vi "Main.vi"(11 "Module Admin":refnum<class "Delacor_lib_QMH_Cloneable Module Admin.lvclass">) -> ()   [LabVIEW 2025, in "Data Log.lvlib"]
doc: "This template is based off of the Queued Message Handler design pattern and the Queued Message Handler project template that ships with LabVIEW.\n\nThe main difference is that the queue is private to this module and communication between modules is performed via Broadcast and Request events.\n\nRequest events are wrapped in public API methods and are handled in the Event Handling Loop (EHL) of this VI. Any module can register for Broadcast events sent by this module. The EHL generates messages based on user interface actions.\n\nThe Message Handling Loop (MHL) processes messages generated by the EHL, or by other messages. The messages are string values, so new messages can be added easily to the Message Cases case structure in the MHL. Each message cluster can also provide an optional value for Message Data, which is a variant that can be converted to whatever message-specific data is required.\n_____\nBased on DQMH Dev Tools: Project Template 7.1.2.1547."
uses:
  Data Log.lvlib
  <vilib>/Delacor/Delacor QMH/Libraries/Message Queue_class/Delacor_lib_QMH_Message Queue.lvclass
  Module Data--cluster.ctl
  <vilib>/Utility/miscctls.llb/LVPointTypeDef.ctl
  <vilib>/Delacor/Delacor QMH/Libraries/Message Queue_class/Delacor_lib_QMH_Enqueue Message (Single).vi
  Stop Argument--cluster.ctl
  <vilib>/Delacor/Delacor QMH/Libraries/Cloneable Module Admin_class/Delacor_lib_QMH_Cloneable Module Admin.lvclass
  Write to .csv (Reply Payload)--cluster.ctl
  Write to .csv Argument--cluster.ctl
  Classes/Data Log/Data Log.lvclass
  Append data (Reply Payload)--cluster.ctl
  Append data Argument--cluster.ctl
panel:
  out "error out":errorcluster
  out "Status":string
  in  "Simulate EHL Error":bool
  in  "Simulate MHL Error":bool
  # "Other processes communicate with this Module via its Public API (wrappers for its Request Events).\n\nThis Module communicates with other processes via its Broadcast Events.\nAny process that wants to receive these messages can register for this module's Broadcast events."
  # "This template is for the DQMH framework. See the block diagram for more information on how to use this template."
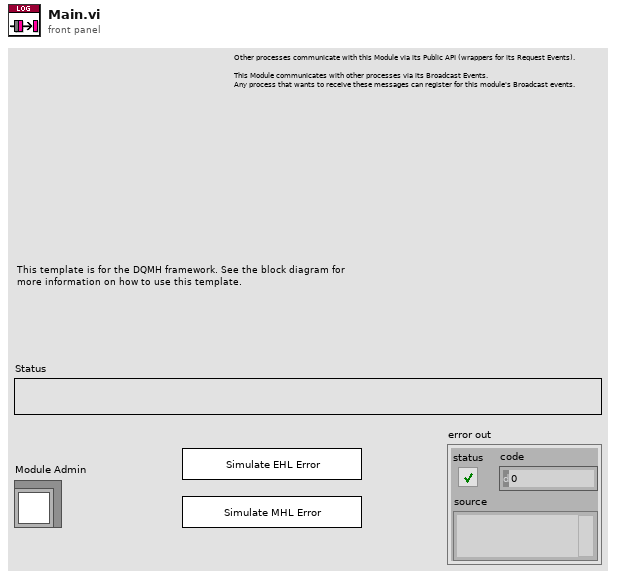
[diagram p1: front panel]
types:
  T1 = typedef "Data Log.lvlib/Request Events--cluster.ctl" = cluster{"Stop Module":refnum<user-event>, "Show Panel":refnum<user-event>, "Hide Panel":refnum<user-event>, "Show Diagram":refnum<user-event>, "Get Module Execution Status":refnum<user-event>, "Write to .csv":refnum<user-event>, "Append data":refnum<user-event>}
  T2 = typedef "Data Log.lvlib/Module Data--cluster.ctl" = cluster{"Status":string, "Data Log Object":refnum<class "Data Log.lvclass">}
  T3 = enum32{"invalid lock state", "Not Locked", "Locked (No Password)", "Password-protected"}
  T4 = typedef "Data Log.lvlib/Stop Argument--cluster.ctl" = cluster{"Module ID":i32, "Origin":string, "Exit via Stop Module Req?":bool, "Wait for Module to stop?":bool}
  T5 = typedef "Data Log.lvlib/Write to .csv Argument--cluster.ctl" = cluster{"Module ID":i32, "csv path":path, "Wait Notifier":refnum<notifier>, "wait for reply":bool}
  T6 = typedef "Data Log.lvlib/Append data Argument--cluster.ctl" = cluster{"Module ID":i32, "Time Stamp":timestamp, "Array":dbl[], "Wait Notifier":refnum<notifier>, "wait for reply":bool}
  T7 = typedef "LVPointTypeDef.ctl" = cluster{"Horizontal":i16, "Vertical":i16}
  T8 = enum32{"Invalid", "Standard", "Closed", "Hidden", "Minimized", "Maximized"}
  T9 = typedef "Data Log.lvlib/Write to .csv (Reply Payload)--cluster.ctl" = cluster{"Module ID":i32, "error":errorcluster}
  T10 = typedef "Data Log.lvlib/Append data (Reply Payload)--cluster.ctl" = cluster{"Module ID":i32, "error":errorcluster}
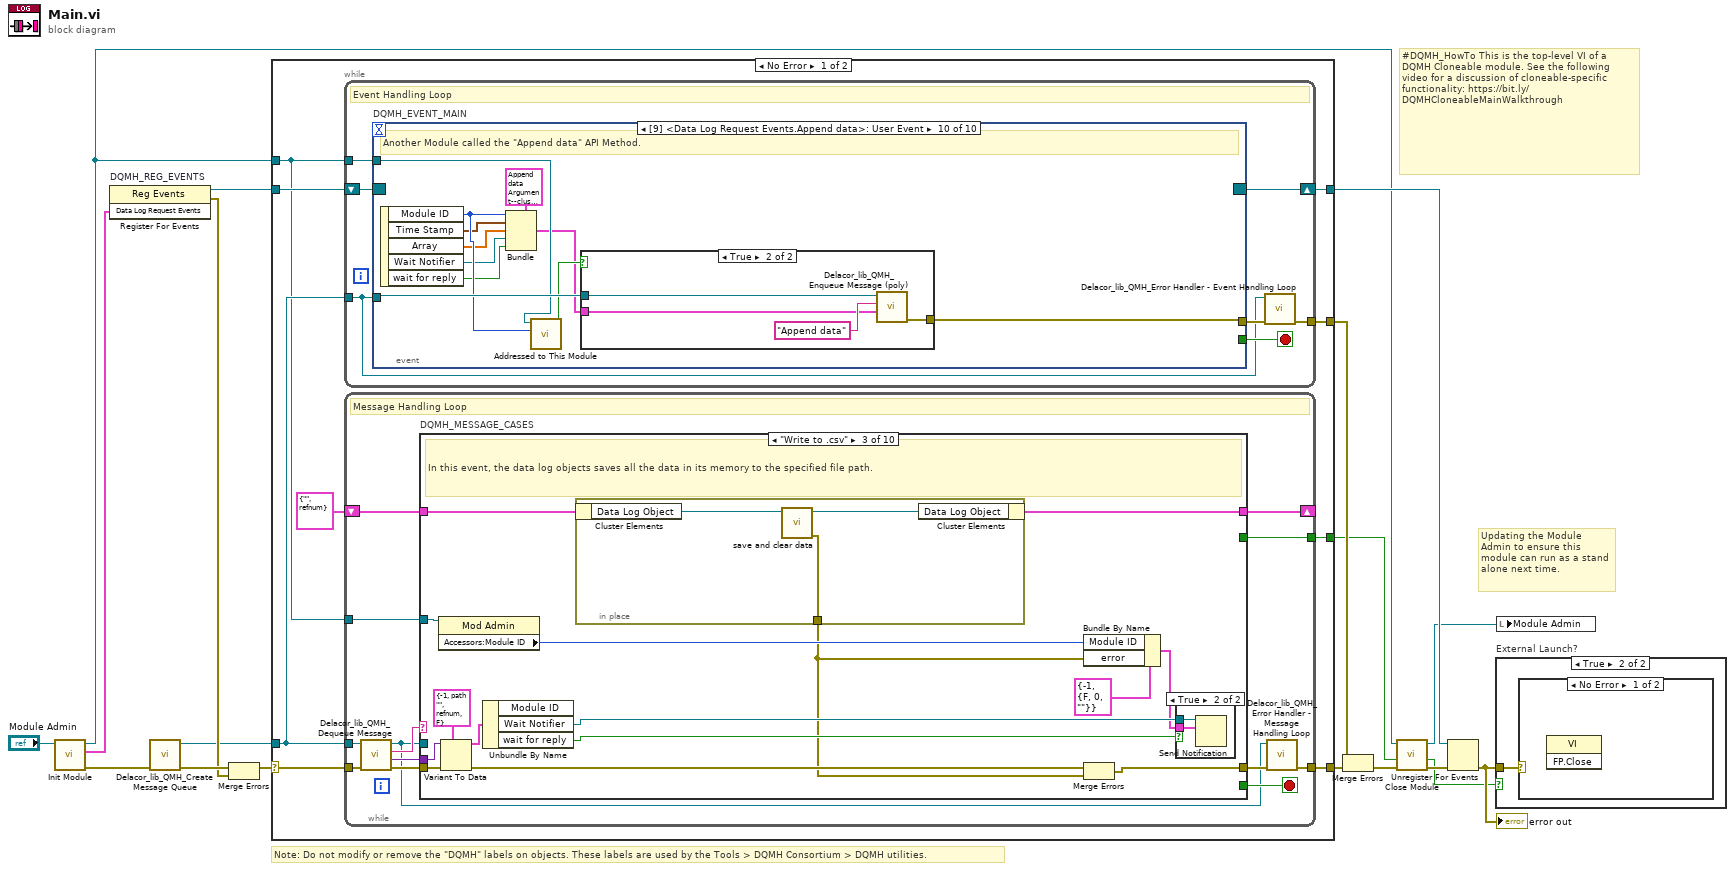
[diagram p0: block diagram]
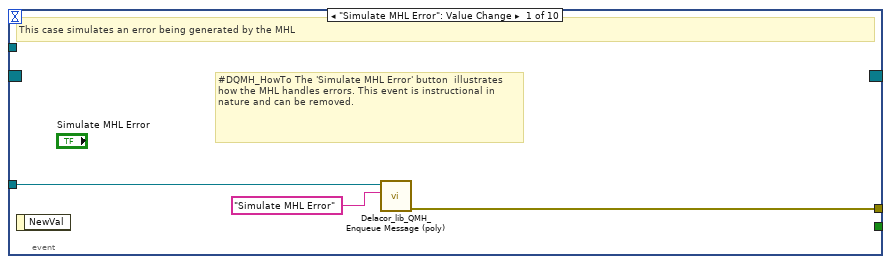
[diagram p2: hidden frame]
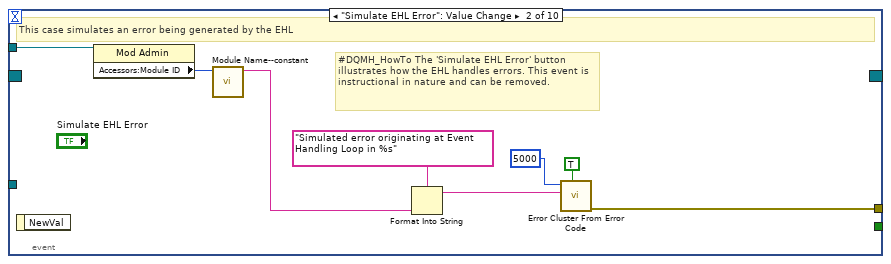
[diagram p3: hidden frame]
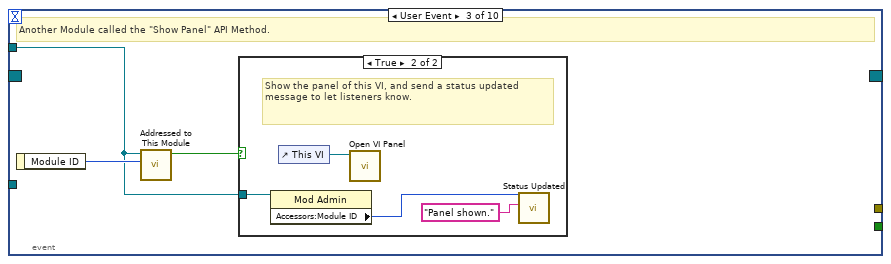
[diagram p4: hidden frame]
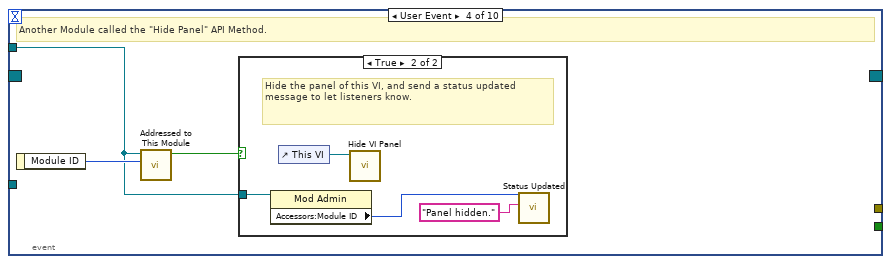
[diagram p6: hidden frame]
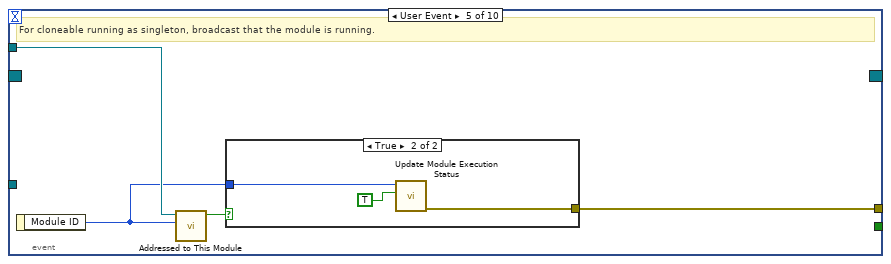
[diagram p8: hidden frame]
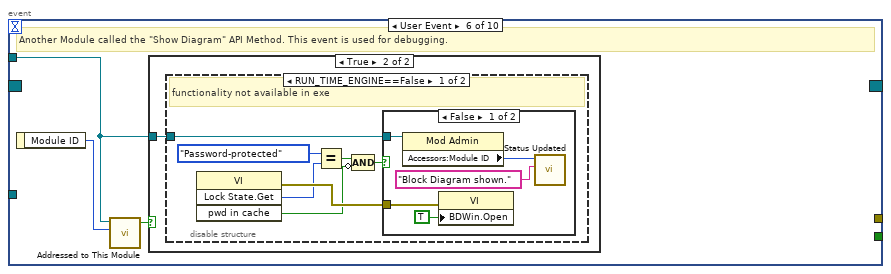
[diagram p10: hidden frame]
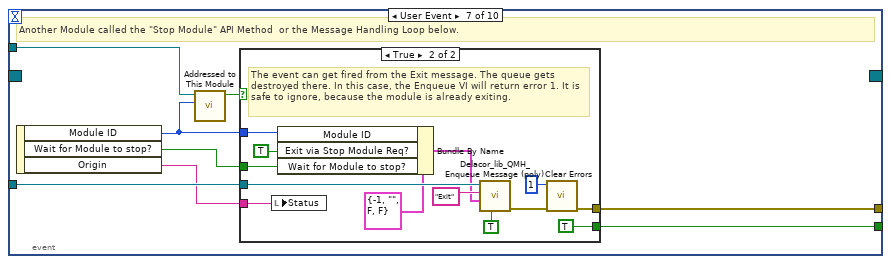
[diagram p14: hidden frame]
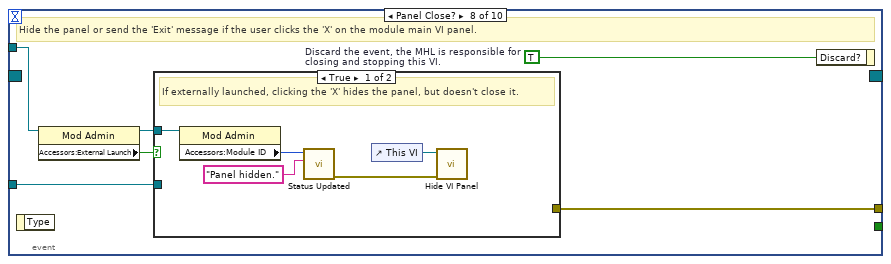
[diagram p16: hidden frame]
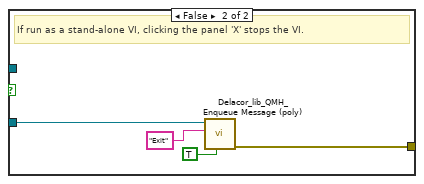
[diagram p17: hidden frame]
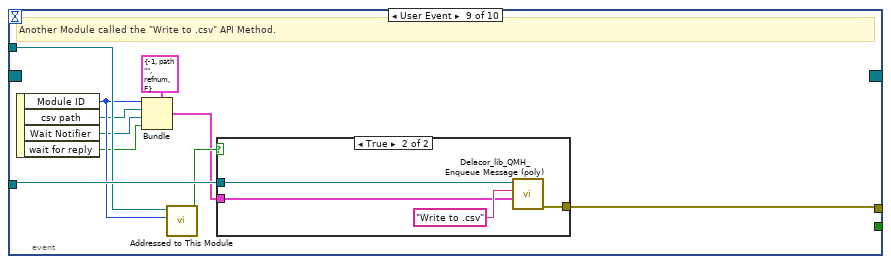
[diagram p18: hidden frame]
diagram:
  # "#DQMH_HowTo This is the top-level VI of a DQMH Cloneable module. See the following video for a discussion of cloneable-specific functionality: https://bit.ly/DQMHCloneableMainWalkthrough"
  # "Note: Do not modify or remove the \"DQMH\" labels on objects. These labels are used by the Tools > DQMH Consortium > DQMH utilities."
  # "Updating the Module Admin to ensure this module can run as a stand alone next time."
  n1 = call "Init Module.vi"("Cloneable Module Admin in"="Module Admin") -> ("error out"=w15:errorcluster, "Data Log Request Events"=w7:T1, "Cloneable Module Admin out"=w4:refnum<class "Delacor_lib_QMH_Cloneable Module Admin.lvclass">)  [unwired: 8 in]
  n2 = register-events "DQMH_REG_EVENTS"(w7) -> (reference out=w8:refnum<event-registration>, error out=w10:errorcluster)  [unwired: 2 in]
  n3 = call <vilib>:"Delacor_lib_QMH_Create Message Queue.vi"("error in"=w15) -> ("error out"=w12:errorcluster, "Message Queue"=w6:refnum<class "Delacor_lib_QMH_Message Queue.lvclass">)  [unwired: 9 in]
  n4 = Merge Errors(w12, w10) -> (w11:errorcluster)
  n5 = case shown="No Error" w11 {
    selector: w11 -> [w25 w300]
    tunnel: [w27 w299] -> w16
    tunnel: [w24 w298] -> w9
    tunnel: w8 -> [w22 w298]
    tunnel: w6 -> [w21 w291]
    tunnel: [w26 _] -> w17
    tunnel: w4 -> [w20 w294]
    tunnel: [w19 _] -> w2
    frame No Error {
      n6 = while {
        tunnel: w21 -> [w28]
        shift-right: [w31] -> w24
        shift-left: w22 -> [w32]
        tunnel: [w33] -> w26
        tunnel: w20 -> [w29]
        stop <- w30 stop-if-true
        # "Event Handling Loop"
        n7 = event "DQMH_EVENT_MAIN" shown="[9] <Data Log Request Events.Append data>: User Event" {
          selector: w32 -> [_ _ _ _ _ _ _ _ _ _]
          dyn-events: [_ _ _ _ _ _ _ _ _ _] -> w31
          timeout: _ -> [_ _ _ _ _ _ _ _ _ _]
          tunnel: [_ _ _ _ _ _ w86 _ _ _] -> w30
          tunnel: w28 -> [w36 _ _ _ _ _ w89 w106 w128 w143]
          tunnel: [w37 w45 _ _ w63 _ w90 w109 w119 w133] -> w34
          tunnel: w29 -> [_ w44 w46 w53 w61 w67 w88 w107 w126 w141]
          event "Simulate MHL Error": Value Change {
            # "#DQMH_HowTo The 'Simulate MHL Error' button  illustrates how the MHL handles errors. This event is instructional in nature and can be removed."
            # "This case simulates an error being generated by the MHL"
            n8 = event-data() -> ()  [unwired: 1 in, 1 out]
            n9 = call-poly <vilib>:"Delacor_lib_QMH_Enqueue Message (poly).vi"("Message"="Simulate MHL Error", "Message Queue in"=w36) -> ("error out"=w37:errorcluster)  [unwired: 8 in, 1 out]
          }
          event "Simulate EHL Error": Value Change {
            # "#DQMH_HowTo The 'Simulate EHL Error' button  illustrates how the EHL handles errors. This event is instructional in nature and can be removed."
            # "This case simulates an error being generated by the EHL"
            n10 = event-data() -> ()  [unwired: 1 in, 1 out]
            n11 = property on="Property Node" class="Mod Admin"(reference=w44) -> ("Accessors:Module ID"=w43:i32)  [unwired: 1 in, 2 out]
            n12 = call "Module Name--constant.vi"("Module ID"=w43) -> ("Module Name"=w38:string)  [unwired: 10 in]
            n13 = Format Into String(format string="Simulated error originating at Event Handling Loop in %s", w38) -> (resulting string=w41:string)  [unwired: 2 in, 1 out]
            n14 = call <vilib>:"Error Cluster From Error Code.vi"("show call chain? (False)"=TRUE, "error message (\"\")"=w41, "error code (0)"=5000) -> ("error out"=w45:errorcluster)  [unwired: 6 in]
          }
          event User Event {
            # "Another Module called the \"Show Panel\" API Method."
            n15 = event-data() -> ("Module ID"=w47:i32)  [unwired: 1 in]
            n16 = call "Addressed to This Module.vi"("Module ID from Argument"=w47, "Module Admin"=w46) -> ("Addressed to this instance?"=w48:bool)  [unwired: 8 in, 1 out]
            n17 = case shown="True" w48 {
              tunnel: w46 -> [_ w50]
              frame False {
              }
              frame True {
                # "Show the panel of this VI, and send a status updated message to let listeners know."
                n18 = property on="Property Node" class="Mod Admin"(reference=w50) -> ("Accessors:Module ID"=w49:i32)  [unwired: 1 in, 2 out]
                n19 = control-ref of="This VI"() -> (w52:refnum<vi>)
                n20 = call "Open VI Panel.vi"("VI"=w52) -> ()  [unwired: 10 in, 1 out]
                n21 = call "Status Updated.vi"("Status"="Panel shown." ("format string"), "Module ID"=w49) -> ()  [unwired: 9 in, 1 out]
              }
            }
          }
          event User Event {
            # "Another Module called the \"Hide Panel\" API Method."
            n22 = event-data() -> ("Module ID"=w54:i32)  [unwired: 1 in]
            n23 = call "Addressed to This Module.vi"("Module ID from Argument"=w54, "Module Admin"=w53) -> ("Addressed to this instance?"=w55:bool)  [unwired: 8 in, 1 out]
            n24 = case shown="True" w55 {
              tunnel: w53 -> [_ w57]
              frame False {
              }
              frame True {
                # "Hide the panel of this VI, and send a status updated message to let listeners know."
                n25 = property on="Property Node" class="Mod Admin"(reference=w57) -> ("Accessors:Module ID"=w56:i32)  [unwired: 1 in, 2 out]
                n26 = control-ref of="This VI"() -> (w59:refnum<vi>)
                n27 = call "Hide VI Panel.vi"("VI"=w59) -> ()  [unwired: 10 in, 1 out]
                n28 = call "Status Updated.vi"("Status"="Panel hidden." ("format string"), "Module ID"=w56) -> ()  [unwired: 9 in, 1 out]
              }
            }
          }
          event User Event {
            # "For cloneable running as singleton, broadcast that the module is running."
            n29 = event-data() -> ("Module ID"=w60:i32)  [unwired: 1 in]
            n30 = call "Addressed to This Module.vi"("Module ID from Argument"=w60, "Module Admin"=w61) -> ("Addressed to this instance?"=w62:bool)  [unwired: 8 in, 1 out]
            n31 = case shown="True" w62 {
              tunnel: [_ w66] -> w63
              tunnel: w60 -> [_ w65]
              frame False {
              }
              frame True {
                n32 = call "Update Module Execution Status.vi"("Running?"=TRUE, "Module ID"=w65) -> ("error out"=w66:errorcluster)  [unwired: 9 in]
              }
            }
          }
          event User Event {
            # "Another Module called the \"Show Diagram\" API Method. This event is used for debugging."
            n33 = event-data() -> ("Module ID"=w68:i32)  [unwired: 1 in]
            n34 = call "Addressed to This Module.vi"("Module ID from Argument"=w68, "Module Admin"=w67) -> ("Addressed to this instance?"=w69:bool)  [unwired: 8 in, 1 out]
            n35 = case shown="True" w69 {
              tunnel: w67 -> [_ w70]
              frame False {
              }
              frame True {
                n36 = disable-structure shown="RUN_TIME_ENGINE==False" {
                  disable-tunnel: w70 -> [w71 _]
                  frame condition #0 (active) {
                    # "functionality not available in exe"
                    n37 = invoke on="Invoke Node" class="VI" method="Lock State.Get"() -> (error out=w77:errorcluster, "Get Lock State"=w76:T3, "pwd in cache"=w73:bool)  [unwired: 4 in, 1 out]
                    n38 = Equal?(x=T3."Password-protected", y=w76) -> (x = y?=w74:bool)
                    n39 = Compound Arithmetic op=AND(w74, invert w73) -> (w72:bool)
                    n40 = case shown="False" w72 {
                      tunnel: w77 -> [w82 _]
                      tunnel: w71 -> [w79 _]
                      frame False {
                        n41 = property on="Property Node" class="Mod Admin"(reference=w79) -> ("Accessors:Module ID"=w78:i32)  [unwired: 1 in, 2 out]
                        n42 = property on="Property Node" class="VI"(error in=w82, "BDWin.Open"=TRUE ("Block Diagram Window:Open")) -> ()  [unwired: 1 in, 2 out]
                        n43 = call "Status Updated.vi"("Status"="Block Diagram shown." ("format string"), "Module ID"=w78) -> ()  [unwired: 9 in, 1 out]
                      }
                      frame True {
                        # "Password-protected VI, and the password is not in the cache. Do not show the diagram."
                      }
                    }
                  }
                  frame condition #1 {
                  }
                }
              }
            }
          }
          event User Event {
            # "Another Module called the \"Stop Module\" API Method  or the Message Handling Loop below."
            n44 = event-data() -> ("Module ID"=w84:i32, "Wait for Module to stop?"=w85:bool, "Origin"=w83:string)  [unwired: 1 in]
            n45 = call "Addressed to This Module.vi"("Module ID from Argument"=w84, "Module Admin"=w88) -> ("Addressed to this instance?"=w87:bool)  [unwired: 8 in, 1 out]
            n46 = case shown="True" w87 {
              tunnel: [_ w102] -> w90
              tunnel: w89 -> [_ w98]
              tunnel: [_ TRUE] -> w86
              tunnel: w85 -> [_ w93]
              tunnel: w84 -> [_ w95]
              tunnel: w83 -> [_ w91]
              frame False {
              }
              frame True {
                # "The event can get fired from the Exit message. The queue gets destroyed there. In this case, the Enqueue VI will return error 1. It is safe to ignore, because the module is already exiting."
                n47 = local write "Status"(w91) -> ()
                n48 = Bundle By Name(cluster=T4 {"Module ID"=-1, "Origin"="", "Exit via Stop Module Req?"=FALSE, "Wait for Module to stop?"=FALSE} ("Stop Argument"), "Module ID"=w95, "Exit via Stop Module Req?"=TRUE, "Wait for Module to stop?"=w93) -> (w92:T4)
                n49 = call-poly <vilib>:"Delacor_lib_QMH_Enqueue Message (poly).vi"("Priority Message? (F)"=TRUE, "Message Data"=w92, "Message"="Exit", "Message Queue in"=w98) -> ("error out"=w103:errorcluster)  [unwired: 6 in, 1 out]
                n50 = call <vilib>:"Clear Errors.vi"("error in (no error)"=w103, "specific error code to clear (0: all)"=1) -> ("error out"=w102:errorcluster)  [unwired: 4 in, 1 out]
              }
            }
          }
          event Panel Close? {
            w108 = TRUE  # Discard the event, the MHL is responsible for closing and stopping this VI.
            # "Hide the panel or send the 'Exit' message if the user clicks the 'X' on the module main VI panel."
            n51 = event-data() -> ()  [unwired: 1 in, 1 out]
            n52 = property on="Property Node" class="Mod Admin"(reference=w107) -> (reference out=w104:refnum<class "Delacor_lib_QMH_Cloneable Module Admin.lvclass">, "Accessors:External Launch"=w105:bool)  [unwired: 1 in, 1 out]
            n53 = case shown="True" w105 {
              tunnel: w106 -> [_ w117]
              tunnel: [_ w118] -> w109
              tunnel: w104 -> [w112 _]
              frame True {
                # "If externally launched, clicking the 'X' hides the panel, but doesn't close it."
                n54 = property on="Property Node" class="Mod Admin"(reference=w112) -> ("Accessors:Module ID"=w111:i32)  [unwired: 1 in, 2 out]
                n55 = call "Status Updated.vi"("Status"="Panel hidden." ("format string"), "Module ID"=w111) -> ("error out"=w110:errorcluster)  [unwired: 9 in]
                n56 = control-ref of="This VI"() -> (w114:refnum<vi>)
                n57 = call "Hide VI Panel.vi"("error in"=w110, "VI"=w114) -> ()  [unwired: 9 in, 1 out]
              }
              frame False {
                # "If run as a stand-alone VI, clicking the panel 'X' stops the VI."
                n58 = call-poly <vilib>:"Delacor_lib_QMH_Enqueue Message (poly).vi"("Priority Message? (F)"=TRUE, "Message"="Exit", "Message Queue in"=w117) -> ("error out"=w118:errorcluster)  [unwired: 7 in, 1 out]
              }
            }
            n59 = event-data ("Event Filter Node")("Discard?"=w108) -> ()  [unwired: 1 in, 1 out]
          }
          event User Event {
            # "Another Module called the \"Write to .csv\" API Method."
            n60 = event-data() -> ("Module ID"=w123:i32, "csv path"=w122:path, "Wait Notifier"=w121:refnum<notifier>, "wait for reply"=w120:bool)  [unwired: 1 in]
            n61 = Bundle(cluster=T5 {"Module ID"=-1, "csv path"=path "", "Wait Notifier"=refnum, "wait for reply"=FALSE} ("Write to .csv Argument"), "Module ID"=w123, "csv path"=w122, "Wait Notifier"=w121, "wait for reply"=w120) -> (w124:T5)
            n62 = call "Addressed to This Module.vi"("Module ID from Argument"=w123, "Module Admin"=w126) -> ("Addressed to this instance?"=w127:bool)  [unwired: 8 in, 1 out]
            n63 = case shown="True" w127 {
              tunnel: w128 -> [_ w132]
              tunnel: w124 -> [_ w130]
              tunnel: [_ w129] -> w119
              frame False {
              }
              frame True {
                n64 = call-poly <vilib>:"Delacor_lib_QMH_Enqueue Message (poly).vi"("Message Data"=w130, "Message"="Write to .csv", "Message Queue in"=w132) -> ("error out"=w129:errorcluster)  [unwired: 7 in, 1 out]
              }
            }
          }
          event User Event {
            # "Another Module called the \"Append data\" API Method."
            n65 = event-data() -> ("Module ID"=w138:i32, "Time Stamp"=w137:timestamp, "Array"=w136:dbl[], "Wait Notifier"=w135:refnum<notifier>, "wait for reply"=w134:bool)  [unwired: 1 in]
            n66 = Bundle(cluster=T6 {"Module ID"=-1, "Time Stamp"=timestamp(0 s since 1904-01-01), "Array"=[], "Wait Notifier"=refnum, "wait for reply"=FALSE} ("Append data Argument"), "Module ID"=w138, "Time Stamp"=w137, "Array"=w136, "Wait Notifier"=w135, "wait for reply"=w134) -> (w139:T6)
            n67 = call "Addressed to This Module.vi"("Module ID from Argument"=w138, "Module Admin"=w141) -> ("Addressed to this instance?"=w142:bool)  [unwired: 8 in, 1 out]
            n68 = case shown="True" w142 {
              tunnel: w143 -> [_ w147]
              tunnel: w139 -> [_ w145]
              tunnel: [_ w144] -> w133
              frame False {
              }
              frame True {
                n69 = call-poly <vilib>:"Delacor_lib_QMH_Enqueue Message (poly).vi"("Message Data"=w145, "Message"="Append data", "Message Queue in"=w147) -> ("error out"=w144:errorcluster)  [unwired: 7 in, 1 out]
              }
            }
          }
        }
        n70 = call-dynamic "Delacor_lib_QMH_Error Handler - Event Handling Loop.vi"("error in"=w34, "Message Queue in"=w28) -> ("dup error in"=w33:errorcluster)  [unwired: 8 in, 1 out]
      }
      n71 = while {
        tunnel: w21 -> [w148]
        shift-right: [w155] -> _
        shift-left: T2 {"Status"="", "Data Log Object"=refnum} ("Data Cluster") -> [w156]
        tunnel: w25 -> [w159]
        tunnel: [w157] -> w27
        tunnel: w20 -> [w150]
        tunnel: [w149] -> w19
        stop <- w154 stop-if-true
        # "Message Handling Loop"
        n72 = call-dynamic "Delacor_lib_QMH_Dequeue Message.vi"("error in"=w159, "Message Queue in"=w148) -> ("error out"=w158:errorcluster, "Message Data"=w152:variant, "Message"=w153:string, "Message Queue out"=w151:refnum<class "Delacor_lib_QMH_Message Queue.lvclass">)  [unwired: 6 in]
        n73 = case "DQMH_MESSAGE_CASES" shown="\"Write to .csv\"" w153 {
          selector: w153 -> [_ _ _ _ _ _ _ _ _ w280]
          tunnel: w151 -> [_ _ _ _ _ _ w235 _ w272 _]
          tunnel: w158 -> [w179 w183 w198 w220 w230 w232 w244 w261 w278 w289]
          tunnel: [w177 w183 w189 w211 w229 w232 w240 w260 w273 w290] -> w160
          tunnel: w156 -> [w170 w182 w186 w208 w228 w231 w239 w258 w271 w287]
          tunnel: [w169 w182 w185 w207 w228 w231 w239 w258 w271 w287] -> w155
          tunnel: [_ _ _ _ _ _ _ _ w270 _] -> w154
          tunnel: w152 -> [_ _ w196 w218 _ _ w238 _ w268 _]
          tunnel: w150 -> [w165 _ w187 w209 _ _ w237 w256 w263 w286]
          tunnel: [_ _ _ _ _ _ _ _ w266 _] -> w149
          frame "Initialize" {
            w162 = "Initial Message" ("Initial Message")
            # "#DQMH_CodeNeeded - Initialize the appearance of the front panel."
            # "#DQMH_CodeNeeded - Initialize your state data here."
            # "Initialize - Any operation that needs to be done before the module can receive messages. Synchronize Caller Events.vi will inform Start Module.vi that the module has launched and is ready to receive messages. Module Did Init.vi will broadcast that the module initialized."
            n74 = call "Synchronize Caller Events.vi"("error in"=w179, "Module Admin"=w165) -> ("error out"=w178:errorcluster, "Module Admin out"=w164:refnum<class "Delacor_lib_QMH_Cloneable Module Admin.lvclass">)  [unwired: 8 in]
            n75 = property on="Property Node" class="Mod Admin"(reference=w164) -> ("Accessors:Module ID"=w161:i32, "Accessors:External Launch"=w166:bool)  [unwired: 1 in, 2 out]
            n76 = call "Module Name--constant.vi"("Module ID"=w161) -> ("Module Name"=w174:string)  [unwired: 10 in]
            n77 = property on="Property Node" class="VI"("Front Panel.Title"=w174) -> (reference out=w176:refnum<vi>, error out=w181:errorcluster)  [unwired: 2 in]
            n78 = Select(t=T8."Hidden" ("State"), s=w166, f=T8."Standard" ("State")) -> (s? t:f=w171:T8)
            n79 = invoke on="Invoke Node" class="VI" method="FP.Open"(reference=w176, error in=w181, "State"=w171) -> (reference out=w175:refnum<vi>, error out=w180:errorcluster)  [unwired: 2 in, 3 out]
            n80 = Bundle By Name(cluster=w170, "Status"=w162) -> (w169:T2)
            n81 = invoke on="Invoke Node" class="VI" method="FP.Center"(reference=w175, error in=w180) -> ()  [unwired: 1 in, 3 out]
            n82 = property on="Pane" class="Pane"("Origin"=T7 {"Horizontal"=0, "Vertical"=0}) -> ()  [unwired: 2 in, 2 out]
            n83 = call "Module Name--constant.vi"("Module ID"=w161) -> ("Module Name"=w167:string)  [unwired: 10 in]
            n84 = call "Module Did Init.vi"("error in"=w178, "Initialized?"=TRUE, "Origin"=w167, "Module ID"=w161) -> ("error out"=w177:errorcluster)  [unwired: 7 in]
            "Status" <- w162
          }
          frame "---Module Specific---" {
            # "Separator -- The following cases handle messages specific to this Module."
          }
          frame "Write to .csv" {
            # "In this event, the data log objects saves all the data in its memory to the specified file path."
            n85 = property class="Mod Admin"(reference=w187) -> ("Accessors:Module ID"=w188:i32)  [unwired: 1 in, 2 out]
            n86 = Variant To Data(error in=w198, type=T5 {"Module ID"=-1, "csv path"=path "", "Wait Notifier"=refnum, "wait for reply"=FALSE} ("Write to .csv Argument"), Variant=w196) -> (data=w194:T5, error out=w197:errorcluster)
            n87 = Unbundle By Name(w194) -> ("Wait Notifier"=w193:refnum<notifier>, "wait for reply"=w192:bool)  [unwired: 1 out]
            n88 = in-place {
              in-place-border: [w199] -> w184
              n89 = in-place-cluster #1(w186) -> ("Data Log Object"=w201:refnum<class "Data Log.lvclass">)
              n90 = call-dynamic "save and clear data.vi"("Data Log in"=w201) -> ("error out"=w199:errorcluster, "Data Log out"=w200:refnum<class "Data Log.lvclass">)  [unwired: 9 in]
              n91 = in-place-cluster #1("Data Log Object"=w200) -> (w185:T2)
            }
            n92 = Bundle By Name(cluster=T9 {"Module ID"=-1, "error"={"status"=FALSE, "code"=0, "source"=""}} ("Write to .csv (Reply Payload)"), "Module ID"=w188, "error"=w184) -> (w191:T9)
            n93 = Merge Errors(w197, w184) -> (w189:errorcluster)
            n94 = case "DQMH_FIRE_NOTIFIER" shown="True" w192 {
              tunnel: w193 -> [_ w203]
              tunnel: w191 -> [_ w202]
              frame False {
              }
              frame True {
                n95 = Send Notification(notification=w202, notifier=w203) -> ()  [unwired: 1 in, 2 out]
              }
            }
          }
          frame "Append data" {
            # "Adds specified data to end of array"
            n96 = property class="Mod Admin"(reference=w209) -> ("Accessors:Module ID"=w210:i32)  [unwired: 1 in, 2 out]
            n97 = Variant To Data(error in=w220, type=T6 {"Module ID"=-1, "Time Stamp"=timestamp(0 s since 1904-01-01), "Array"=[], "Wait Notifier"=refnum, "wait for reply"=FALSE} ("Append data Argument"), Variant=w218) -> (data=w216:T6, error out=w219:errorcluster)
            n98 = Unbundle By Name(w216) -> ("Time Stamp"=w206:timestamp, "Array"=w205:dbl[], "Wait Notifier"=w215:refnum<notifier>, "wait for reply"=w214:bool)  [unwired: 1 out]
            n99 = in-place {
              in-place-border: w206 -> [w223]
              in-place-border: w205 -> [w222]
              in-place-border: [w221] -> w204
              n100 = in-place-cluster #2(w208) -> ("Data Log Object"=w225:refnum<class "Data Log.lvclass">)
              n101 = call-dynamic "append data.vi"("Array"=w222, "Time Stamp"=w223, "Data Log in"=w225) -> ("error out"=w221:errorcluster, "Data Log out"=w224:refnum<class "Data Log.lvclass">)  [unwired: 7 in]
              n102 = in-place-cluster #2("Data Log Object"=w224) -> (w207:T2)
            }
            n103 = Bundle By Name(cluster=T10 {"Module ID"=-1, "error"={"status"=FALSE, "code"=0, "source"=""}} ("Append data (Reply Payload)"), "Module ID"=w210, "error"=w204) -> (w213:T10)
            n104 = Merge Errors(w219, w204) -> (w211:errorcluster)
            n105 = case "DQMH_FIRE_NOTIFIER" shown="True" w214 {
              tunnel: w215 -> [_ w227]
              tunnel: w213 -> [_ w226]
              frame False {
              }
              frame True {
                n106 = Send Notification(notification=w226, notifier=w227) -> ()  [unwired: 1 in, 2 out]
              }
            }
          }
          frame "---Copy This Frame---" {
            # "Duplicate this frame when creating new messages.  Change this comment in the duplicated frame to describe this message."
            n107 = Merge Errors(w230) -> (w229:errorcluster)
          }
          frame "---Exit and Error Handling---" {
            # "Separator - the following cases handle errors and exit messages."
          }
          frame "Error" {
            # "#DQMH_CodeRecommended - If the module is running in standalone mode (External Launch = FALSE), this code will pop up an error dialog and call the 'Exit' message if an error occurs. Add more fine-grained error management here."
            # "Error - Check the error message data and respond accordingly. This message is sent by the \"Error Handler\" VIs at the end of each loop in this application."
            n108 = property on="Property Node" class="Mod Admin"(reference=w237) -> ("Accessors:External Launch"=w236:bool, "Accessors:Module ID"=w234:i32)  [unwired: 1 in, 2 out]
            n109 = Variant To Data(error in=w244, type=errorcluster {"status"=FALSE, "code"=0, "source"=""} ("error constant"), Variant=w238) -> (data=w233:errorcluster, error out=w242:errorcluster)
            n110 = local write "error out"(w233) -> ()
            n111 = call "Error Reported.vi"("Error"=w233, "Module ID"=w234) -> ()  [unwired: 9 in, 1 out]
            n112 = case shown="False" w236 {
              tunnel: [w249 _] -> w241
              tunnel: w235 -> [w247 _]
              tunnel: w233 -> [w248 _]
              frame False {
                n113 = disable-structure shown="Default" {
                  disable-tunnel: w248 -> [w250 _]
                  frame condition #0 (active) {
                    # "If the module is running standalone, then pop up an error dialog and call the \"Exit\" message."
                    n114 = call <vilib>:"Simple Error Handler.vi"("error in (no error)"=w250) -> ()  [unwired: 4 in, 5 out]
                  }
                  frame condition #1 {
                    # "To prevent the Simple Error Handler VI from being loaded (e.g. when deploying to a Real-Time target), add the Conditional Disable Symbol \"DQMH_Disable_SEH\" to your project and set it to TRUE."
                  }
                }
                n115 = call-poly <vilib>:"Delacor_lib_QMH_Enqueue Message (poly).vi"("Priority Message? (F)"=TRUE, "Message"="Exit", "Message Queue in"=w247) -> ("error out"=w249:errorcluster)  [unwired: 7 in, 1 out]
              }
              frame True {
                # "If the module was launched externally, calling the Error Reported broadcast VI is the only action performed by the \"Error\" message. The module's caller can then process the error appropriately."
              }
            }
            n116 = Merge Errors(w242, w241) -> (w240:errorcluster)
          }
          frame "Simulate MHL Error" {
            # "#DQMH_HowTo The 'Simulate MHL Error' button  illustrates how the MHL handles errors. This event is instructional in nature and can be removed."
            # "Simulate an error occurring at the MHL"
            n117 = property on="Property Node" class="Mod Admin"(reference=w256) -> ("Accessors:Module ID"=w257:i32)  [unwired: 1 in, 2 out]
            n118 = call "Module Name--constant.vi"("Module ID"=w257) -> ("Module Name"=w252:string)  [unwired: 10 in]
            n119 = Format Into String(format string="Simulated error originating at Message Handling Loop in %s", w252) -> (resulting string=w253:string)  [unwired: 2 in, 1 out]
            n120 = call <vilib>:"Error Cluster From Error Code.vi"("show call chain? (False)"=TRUE, "error message (\"\")"=w253, "error code (0)"=5001) -> ("error out"=w259:errorcluster)  [unwired: 6 in]
            n121 = Merge Errors(w261, w259) -> (w260:errorcluster)
          }
          frame "Exit" {
            w269 = 91  # 91: not all Exit messages will have an argument
            w270 = TRUE  # Stop the VI
            # "Release the message queue reference"
            # "#DQMH_CodeNeeded - Add any required cleanup code here."
            # "Exit - Exit the application."
            n122 = Variant To Data(error in=w278, type=T4 {"Module ID"=-1, "Origin"="", "Exit via Stop Module Req?"=FALSE, "Wait for Module to stop?"=FALSE} ("Stop Argument"), Variant=w268) -> (data=w265:T4, error out=w274:errorcluster)
            n123 = call <vilib>:"Clear Errors.vi"("error in (no error)"=w274, "specific error code to clear (0: all)"=w269) -> ("error out"=w277:errorcluster)  [unwired: 4 in, 1 out]
            n124 = property on="Property Node" class="Mod Admin"(reference=w263) -> ("Accessors:Module ID"=w262:i32)  [unwired: 1 in, 2 out]
            n125 = control-ref of="This VI"() -> (w264:refnum<vi>)
            n126 = call-dynamic "Delacor_lib_QMH_Release Message Queue.vi"("error in"=w277, "Message Queue"=w272) -> ("error out"=w276:errorcluster)  [unwired: 9 in]
            n127 = call "Handle Exit.vi"("Stop Argument"=w265, "Module Admin in"=w263, "VI reference"=w264) -> ("error out"=w275:errorcluster, "Wait for Stop?"=w266:bool)  [unwired: 7 in]
            n128 = Merge Errors(w276, w275) -> (w273:errorcluster)
            n129 = call "Error Reported.vi"("Error"=w273, "Module ID"=w262) -> ()  [unwired: 9 in, 1 out]
          }
          frame Default {
            # "'Default' case only runs if there is a message that isn't defined in any of the other cases.  Output a programming error."
            n130 = property on="Property Node" class="Mod Admin"(reference=w286) -> ("Accessors:Module ID"=w285:i32)  [unwired: 1 in, 2 out]
            n131 = call "Module Name--constant.vi"("Module ID"=w285) -> ("Module Name"=w279:string)  [unwired: 10 in]
            n132 = Format Into String(format string="The invalid message string \"%s\" was received in the Message Handling Loop for module \"%s\".", w280, w279) -> (resulting string=w282:string)  [unwired: 2 in, 1 out]
            n133 = call <vilib>:"Error Cluster From Error Code.vi"("show call chain? (False)"=TRUE, "error message (\"\")"=w282, "error code (0)"=1) -> ("error out"=w288:errorcluster)  [unwired: 6 in]
            n134 = Merge Errors(w289, w288) -> (w290:errorcluster)
          }
        }
        n135 = call-dynamic "Delacor_lib_QMH_Error Handler - Message Handling Loop.vi"("error in"=w160, "Message Queue in"=w151) -> ("dup error in"=w157:errorcluster)  [unwired: 8 in, 1 out]
      }
    }
    frame Error {
      n136 = call "Synchronize Caller Events.vi"("Module Admin"=w294) -> ("Module Admin out"=w293:refnum<class "Delacor_lib_QMH_Cloneable Module Admin.lvclass">)  [unwired: 9 in, 1 out]
      n137 = property on="Property Node" class="Mod Admin"(reference=w293) -> ("Accessors:Module ID"=w292:i32)  [unwired: 1 in, 2 out]
      n138 = call-dynamic "Delacor_lib_QMH_Release Message Queue.vi"("error in"=w300, "Message Queue"=w291) -> ("error out"=w299:errorcluster)  [unwired: 9 in]
      n139 = call "Module Name--constant.vi"("Module ID"=w292) -> ("Module Name"=w297:string)  [unwired: 10 in]
      n140 = Format Into String(format string="An error occurred during initialization. %s is no longer running.", w297) -> (resulting string=w295:string)  [unwired: 2 in, 1 out]
      n141 = call "Error Reported.vi"("Additional Information"=w295, "Error"=w299, "Module ID"=w292) -> ()  [unwired: 8 in, 1 out]
    }
  }
  n142 = Merge Errors(w17, w16) -> (w18:errorcluster)
  n143 = call "Close Module.vi"("error in"=w18, "Wait for stop?"=w2, "Module Admin in"=w4) -> ("error out"=w14:errorcluster, "External Launch"=w1:bool, "Module Admin out"=w3:refnum<class "Delacor_lib_QMH_Cloneable Module Admin.lvclass">)  [unwired: 6 in]
  n144 = Unregister For Events(event registration refnum=w9, error in=w14) -> (error out=w13:errorcluster)
  "error out" <- w13
  n145 = case "External Launch?" shown="True" w1 {
    tunnel: w13 -> [_ w301]
    frame False {
    }
    frame True {
      n146 = case shown="No Error" w301 {
        frame No Error {
          n147 = invoke class="VI" method="FP.Close"() -> ()  [unwired: 3 in, 3 out]
        }
        frame Error {
          n148 = disable-structure shown="Default" {
            frame condition #0 (active) {
              n149 = invoke class="VI" method="FP.Open"("Activate"=TRUE ("Activate?")) -> ()  [unwired: 4 in, 5 out]
            }
            frame condition #1 {
              # "Don't show panel on error if running inside a built EXE."
            }
          }
        }
      }
    }
  }
  n150 = local write "Module Admin"(w3) -> ()
